vi "Untitled 1.vi"   [LabVIEW 2016, in "Logger.syslog.lvclass"]
uses:
  Logger.syslog.lvclass
  <userlib>/_SEH/Controls/CEH/CEH Actions.ctl
types:
  T1 = typedef "SEH Notification Info.ctl" = cluster{"Priority":i32, "Occurrences":i32, "First Occurrence":timestamp}
  T2 = typedef "CEH Actions.ctl" = enum16{"Log", "Display Error Message", "Safe State", "Shutdown"}
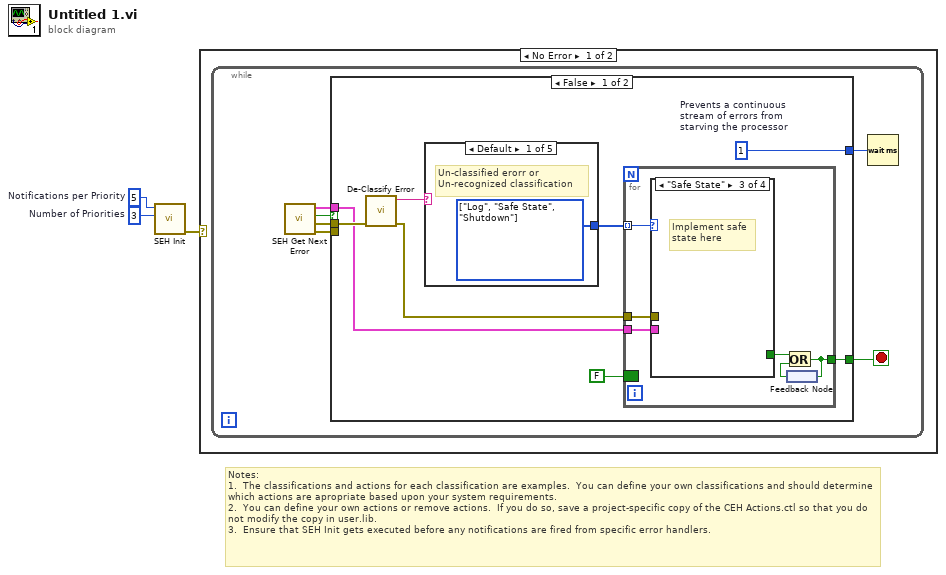
[diagram p0: block diagram]
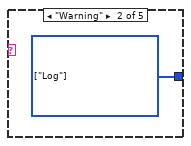
[diagram p2: hidden frame]
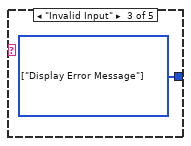
[diagram p3: hidden frame]
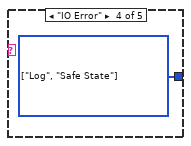
[diagram p4: hidden frame]
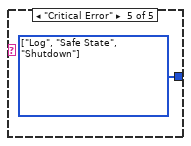
[diagram p5: hidden frame]
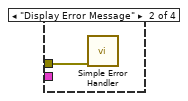
[diagram p7: hidden frame]
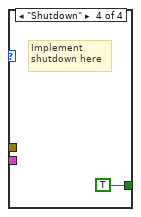
[diagram p8: hidden frame]
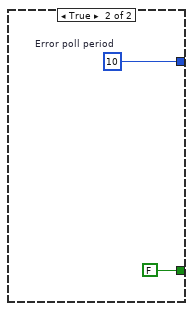
[diagram p9: hidden frame]
diagram:
  w2 = 3  # Number of Priorities
  w1 = 5  # Notifications per Priority
  # "Notes:\n1.  The classifications and actions for each classification are examples.  You can define your own classifications and should determine which actions are apropriate based upon your system requirements.\n2.  You can define your own actions or remove actions.  If you do so, save a project-specific copy of the CEH Actions.ctl so that you do not modify the copy in user.lib.\n3.  Ensure that SEH Init gets executed before any notifications are fired from specific error handlers."
  n1 = call <userlib>:"SEH Init.vi"("Number of Priorities"=w2, "Notifications per Priority"=w1) -> ("error out"=w3:errorcluster)  [unwired: 9 in]
  n2 = case shown="No Error" w3 {
    frame No Error {
      n3 = while {
        stop <- w8 stop-if-true
        n4 = call <userlib>:"SEH Get Next Error.vi"() -> ("Transmission Error"=w4:errorcluster, "Transmitted Error"=w7:errorcluster, "Empty?"=w6:bool, "Notification Info"=w5:T1)  [unwired: 8 in]
        n5 = case shown="False" w6 {
          tunnel: [w17 w32] -> w9
          tunnel: w7 -> [w16 _]
          tunnel: w5 -> [w12 _]
          tunnel: [w11 FALSE] -> w8
          tunnel: w4 -> [_ _]
          frame False {
            w17 = u32 1  # Prevents a continuous stream of errors from starving the processor
            n6 = call <userlib>:"De-Classify Error.vi"("Classified Error"=w16) -> ("De-Classified Error"=w14:errorcluster, "Error Classification"=w15:string)  [unwired: 8 in, 1 out]
            n7 = case shown="Default" w15 {
              tunnel: [w18 w19 w20 w21 w22] -> w13
              frame Default {
                w18 = T2[] [enum."Log", enum."Safe State", enum."Shutdown"] items=["Log", "Display Error Message", "Safe State", "Shutdown"]
                # "Un-classified erorr or\nUn-recognized classification"
              }
              frame "Warning" {
                w19 = T2[] [enum."Log"] items=["Log", "Display Error Message", "Safe State", "Shutdown"]
              }
              frame "Invalid Input" {
                w20 = T2[] [enum."Display Error Message"] items=["Log", "Display Error Message", "Safe State", "Shutdown"]
              }
              frame "IO Error" {
                w21 = T2[] [enum."Log", enum."Safe State"] items=["Log", "Display Error Message", "Safe State", "Shutdown"]
              }
              frame "Critical Error" {
                w22 = T2[] [enum."Log", enum."Safe State", enum."Shutdown"] items=["Log", "Display Error Message", "Safe State", "Shutdown"]
              }
            }
            n8 = for {
              tunnel: w14 -> [w27]
              tunnel: w13 -> [w28] mode=indexing
              tunnel: w12 -> [w26]
              border: FALSE -> [_]
              tunnel: [w23] -> w11
              n9 = case shown="\"Safe State\"" w28 {
                tunnel: w27 -> [_ w29 _ _]
                tunnel: w26 -> [_ _ _ _]
                tunnel: [_ _ _ TRUE] -> w25
                frame "Log", Default {
                  # "Implement log \nhere"
                }
                frame "Display Error Message" {
                  n10 = call <vilib>:"Simple Error Handler.vi"("error in (no error)"=w29) -> ()  [unwired: 4 in, 5 out]
                }
                frame "Safe State" {
                  # "Implement safe\nstate here"
                }
                frame "Shutdown" {
                  # "Implement\nshutdown here"
                }
              }
              n11 = feedback #1() -> (w24:bool)
              n12 = Or(x=w25, y=w24) -> (x .or. y?=w23:bool)
              n13 = feedback-in #1(w23) -> ()
            }
          }
          frame True {
            w32 = u32 10  # Error poll period
          }
        }
        n14 = Wait (ms)(milliseconds to wait=w9) -> ()  [unwired: 1 out]
      }
    }
    frame Error {
      # "Error notification cannot initialize\n(log this)"
    }
  }
